vi "Comsetting.vi"(3 "error in":errorcluster, 4 "Cluster In":T1, 5 "Enum":enum16{"read", "write"}(ring)=enum."write") -> (0 "error our":errorcluster, 1 "Cluster Out":T1, 2 "appended path 2":path)   [LabVIEW 2017]
doc: "VI for saving Hardware setting for PLC IP and Camera IP address. an PORT"
uses:
  <vilib>/Utility/config.llb/Read Key (String).vi
  <vilib>/Utility/config.llb/Write Key (String).vi
  <vilib>/Utility/config.llb/NI_LVConfig.lvlib
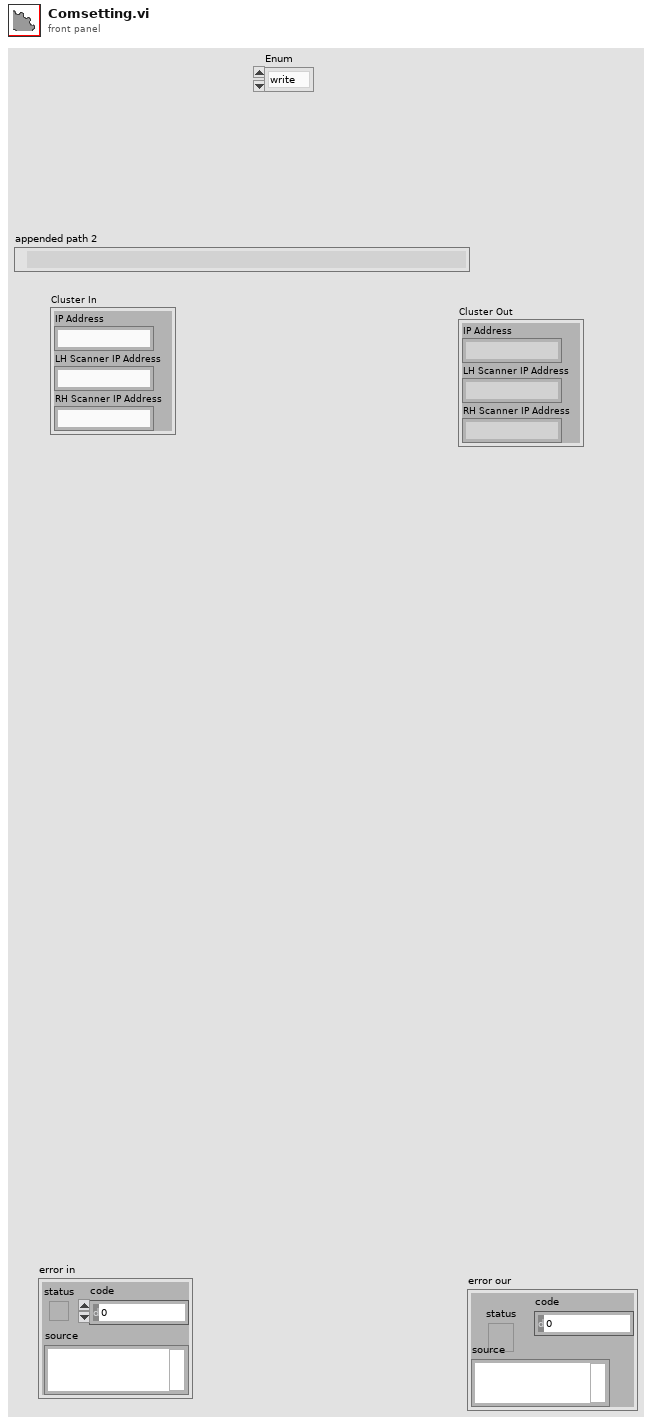
[diagram p1: front panel]
types:
  T1 = cluster{"IP Address":string, "LH Scanner IP Address":string, "RH Scanner IP Address":string}
  T2 = enum32{"invalid app kind", "Development System", "Run Time System", "Student Edition", "Embedded LabVIEW", "Evaluation", "Custom"}
  T3 = typedef "NI_LVConfig.lvlib/Config Data RefNum.ctl" = refnum<k1>
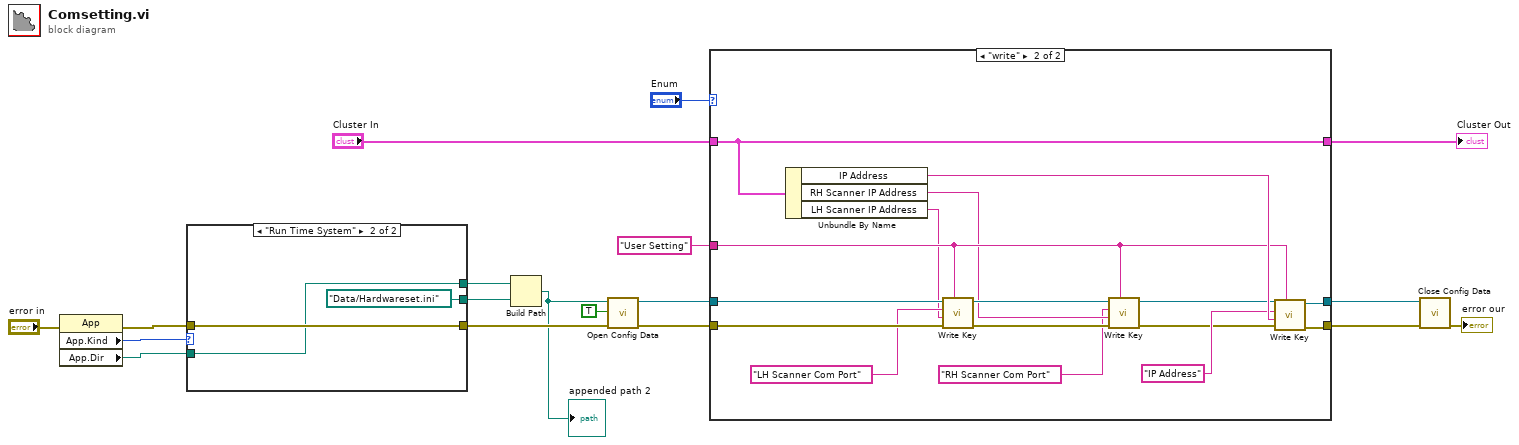
[diagram p0: block diagram]
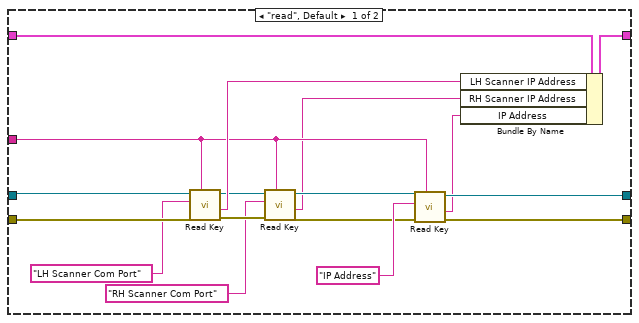
[diagram p2: hidden frame]
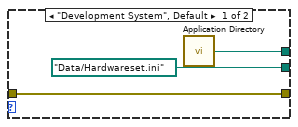
[diagram p3: hidden frame]
diagram:
  n1 = property class="App"(error in="error in") -> (error out=w10:errorcluster, "App.Kind"=w4:T2, "App.Dir"=w9:path)  [unwired: 1 in, 1 out]
  n2 = case shown="\"Run Time System\"" w4 {
    tunnel: [w21 w24] -> w11
    tunnel: w10 -> [w21 w24]
    tunnel: w9 -> [_ w22]
    tunnel: [path "Data/Hardwareset.ini" path "Data/Hardwareset.ini"] -> w8
    tunnel: [w19 w22] -> w7
    frame "Development System", Default {
      n3 = call <vilib>:"Application Directory.vi"() -> ("Application Directory"=w19:path)
    }
    frame "Run Time System" {
    }
  }
  n4 = Build Path(base path=w7, name or relative path=w8) -> (appended path=w6:path)
  "appended path 2" <- w6
  n5 = call <vilib>:"Open Config Data.vi"("error in (no error)"=w11, "create file if necessary (T)"=TRUE, "configuration file path"=w6) -> ("error out"=w17:errorcluster, "refnum"=w16:T3)  [unwired: 6 in, 1 out]
  n6 = case shown="\"write\"" "Enum" {
    tunnel: [w39 w52] -> w14
    tunnel: w17 -> [w37 w56]
    tunnel: w16 -> [w36 w55]
    tunnel: [w38 w51] -> w13
    tunnel: "User Setting" -> [w28 w45]
    tunnel: "Cluster In" -> [w41 w49]
    tunnel: [w40 w49] -> w1
    frame "read", Default {
      n7 = call-poly <vilib>:"Read Key.vi"("section"=w28, "error in (no error)"=w37, "key"="LH Scanner Com Port", "refnum"=w36) -> ("error out"=w29:errorcluster, "value"=w33:string, "refnum out"=w32:T3)  [unwired: 4 in, 1 out]
      n8 = call-poly <vilib>:"Read Key.vi"("section"=w28, "error in (no error)"=w29, "key"="RH Scanner Com Port", "refnum"=w32) -> ("error out"=w30:errorcluster, "value"=w25:string, "refnum out"=w31:T3)  [unwired: 4 in, 1 out]
      n9 = call-poly <vilib>:"Read Key.vi"("section"=w28, "error in (no error)"=w30, "key"="IP Address", "refnum"=w31) -> ("error out"=w39:errorcluster, "value"=w26:string, "refnum out"=w38:T3)  [unwired: 4 in, 1 out]
      n10 = Bundle By Name(cluster=w41, "LH Scanner IP Address"=w33, "RH Scanner IP Address"=w25, "IP Address"=w26) -> (w40:T1)
    }
    frame "write" {
      n11 = Unbundle By Name(w49) -> ("IP Address"=w53:string, "RH Scanner IP Address"=w43:string, "LH Scanner IP Address"=w44:string)
      n12 = call-poly <vilib>:"Write Key.vi"("section"=w45, "error in (no error)"=w56, "value"=w44, "key"="LH Scanner Com Port", "refnum"=w55) -> ("error out"=w57:errorcluster, "refnum out"=w47:T3)  [unwired: 4 in, 1 out]
      n13 = call-poly <vilib>:"Write Key.vi"("section"=w45, "error in (no error)"=w57, "value"=w43, "key"="RH Scanner Com Port", "refnum"=w47) -> ("error out"=w48:errorcluster, "refnum out"=w46:T3)  [unwired: 4 in, 1 out]
      n14 = call-poly <vilib>:"Write Key.vi"("section"=w45, "error in (no error)"=w48, "value"=w53, "key"="IP Address", "refnum"=w46) -> ("error out"=w52:errorcluster, "refnum out"=w51:T3)  [unwired: 4 in, 1 out]
    }
  }
  "Cluster Out" <- w1
  n15 = call <vilib>:"Close Config Data.vi"("error in (no error)"=w14, "refnum"=w13) -> ("error out"=→"error our":errorcluster)  [unwired: 8 in, 1 out]
